vi "Bool_Latch.vi"(6 "Set(t) Reset(f) \nPriority":bool, 7 "Initial State":bool, 8 "Reset":bool, 11 "Set":bool) -> (3 "Output":bool)   [LabVIEW 2020]
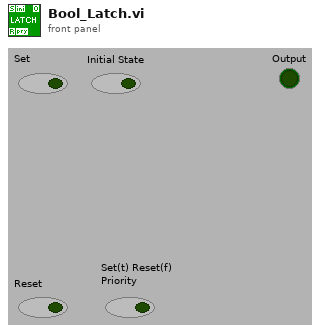
[diagram p1: front panel]
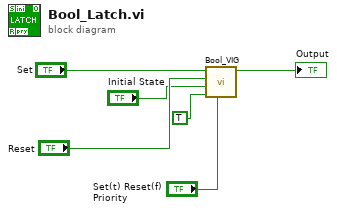
[diagram p0: block diagram]
diagram:
  n1 = call "Bool_VIG.vi"("Set(t) Reset(f) \nDominant"="Set(t) Reset(f) \nPriority", "Latch(t) Edge(f)"=TRUE, "Initial State"="Initial State", "Reset"="Reset", "Input/Set"="Set") -> ("Output"=→"Output":bool)  [unwired: 3 in, 3 out]
